vi "creaRangos.vi"(8 "error in (no error)":errorcluster, 9 "RangoMin":dbl, 10 "ptoCentral":dbl, 11 "RangoMax":dbl) -> (0 "error out":errorcluster, 1 "RangoInf":dbl[](array[numeric]), 2 "RangoSup":dbl[](array[numeric]), 3 "RangoCompleto":dbl[](array[numeric]))   [LabVIEW 2019, in "Prueba06.lvclass"]
uses:
  Prueba06.lvclass
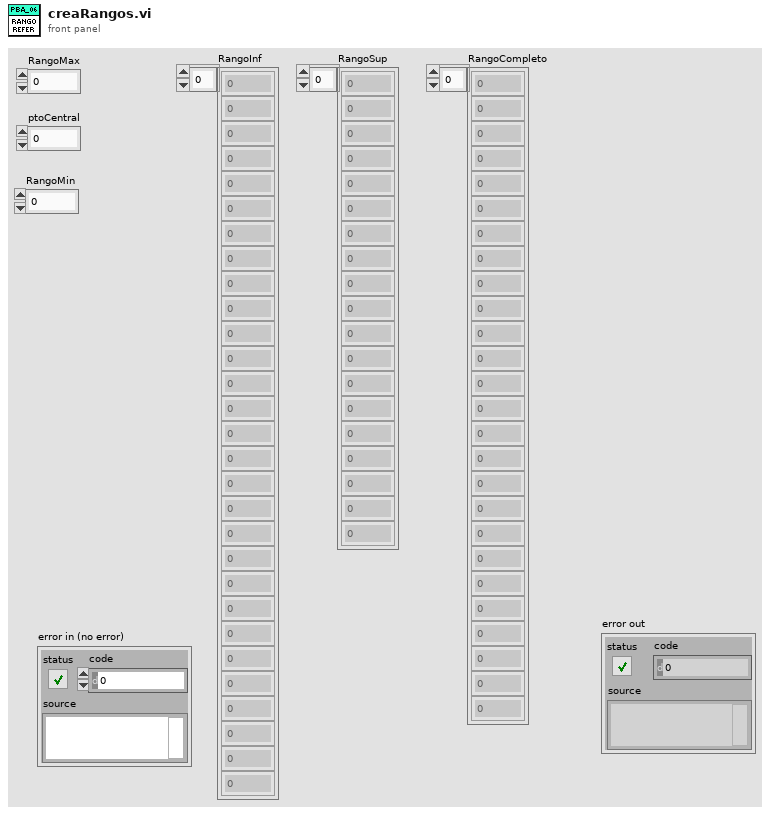
[diagram p1: front panel]
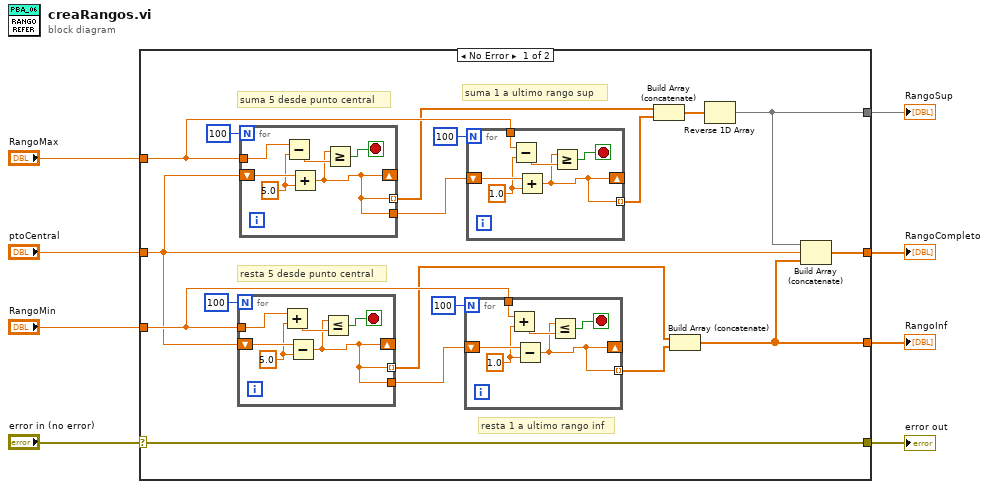
[diagram p0: block diagram]
diagram:
  n1 = case shown="No Error" "error in (no error)" {
    selector: "error in (no error)" -> [w10 w51]
    tunnel: "RangoMax" -> [w26 _]
    tunnel: "RangoMin" -> [w17 _]
    tunnel: [w9 _] -> w6
    tunnel: "ptoCentral" -> [w13 _]
    tunnel: [w12 _] -> w4
    tunnel: [w11 _] -> w3
    tunnel: [w10 w51] -> w1
    frame No Error {
      # "resta 1 a ultimo rango inf"
      # "suma 1 a ultimo rango sup"
      # "resta 5 desde punto central"
      # "suma 5 desde punto central"
      n2 = for {
        N: 100 -> [_]
        tunnel: w17 -> [w36]
        shift-right: [w33] -> _
        shift-left: w13 -> [w38]
        tunnel: [w33] -> w16 mode=indexing
        tunnel: [w33] -> w18
        stop <- w35 stop-if-true
        w37 = 5.0 ("y")
        n3 = Add(x=w36, y=w37) -> (x+y=w34:dbl)
        n4 = Subtract(x=w38, y=w37) -> (x-y=w33:dbl)
        n5 = Less Or Equal?(x=w33, y=w34) -> (x <= y?=w35:bool)
      }
      n6 = for {
        N: 100 -> [_]
        tunnel: w26 -> [w48]
        shift-right: [w45] -> _
        shift-left: w13 -> [w50]
        tunnel: [w45] -> w22 mode=indexing
        tunnel: [w45] -> w25
        stop <- w47 stop-if-true
        w49 = 5.0 ("y")
        n7 = Subtract(x=w48, y=w49) -> (x-y=w46:dbl)
        n8 = Add(x=w50, y=w49) -> (x+y=w45:dbl)
        n9 = Greater Or Equal?(x=w45, y=w46) -> (x >= y?=w47:bool)
      }
      n10 = for {
        N: 100 -> [_]
        shift-right: [w28] -> _
        shift-left: w18 -> [w32]
        tunnel: [w28] -> w15 mode=indexing
        tunnel: w17 -> [w27]
        stop <- w30 stop-if-true
        w31 = 1.0 ("y")
        n11 = Add(x=w27, y=w31) -> (x+y=w29:dbl)
        n12 = Subtract(x=w32, y=w31) -> (x-y=w28:dbl)
        n13 = Less Or Equal?(x=w28, y=w29) -> (x <= y?=w30:bool)
      }
      n14 = for {
        N: 100 -> [_]
        shift-right: [w40] -> _
        shift-left: w25 -> [w44]
        tunnel: [w40] -> w21 mode=indexing
        tunnel: w26 -> [w39]
        stop <- w42 stop-if-true
        w43 = 1.0 ("y")
        n15 = Subtract(x=w39, y=w43) -> (x-y=w41:dbl)
        n16 = Add(x=w44, y=w43) -> (x+y=w40:dbl)
        n17 = Greater Or Equal?(x=w40, y=w41) -> (x >= y?=w42:bool)
      }
      n18 = Build Array (concatenate)(w22, w21) -> (w14:dbl[])
      n19 = Build Array (concatenate)(w16, w15) -> (w12:dbl[])
      n20 = Reverse 1D Array(array=w14) -> (reversed array=w9:dbl[])
      n21 = Build Array (concatenate)(w9, w13, w12) -> (w11:dbl[])
    }
    frame Error {
    }
  }
  "RangoSup" <- w6
  "RangoInf" <- w4
  "error out" <- w1
  "RangoCompleto" <- w3
